vi "write-set.vi"(7 "dvr":refnum<data-value>, 8 "error in (no error)":errorcluster, 10 "y_axis":dbl[][](array[numeric]), 11 "x_axis":dbl[](array[numeric])) -> (0 "error out":errorcluster)   [LabVIEW 2015, in "lv-graph-global.lvlib"]
doc: "Preload can be used to store a data set in total. This can be used to \"load\" data from an alternate source rather than generating a set of points at a time."
uses:
  _controls/data.ctl
  _controls/configuration.ctl
  _controls/store_method.ctl
  lv-graph-global.lvlib
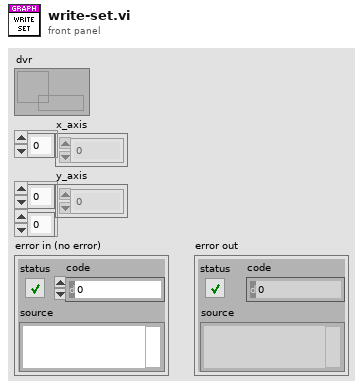
[diagram p1: front panel]
types:
  T1 = typedef "lv-graph-global.lvlib/data.ctl" = cluster{"configuration":T2, "index":i32, "x_axis":dbl[], "y_axis":dbl[][]}
  T2 = typedef "lv-graph-global.lvlib/configuration.ctl" = cluster{"store_method":T3, "rows":i32, "columns":i32}
  T3 = typedef "lv-graph-global.lvlib/store_method.ctl" = enum16{"<store_method>", "fixed", "grow"}
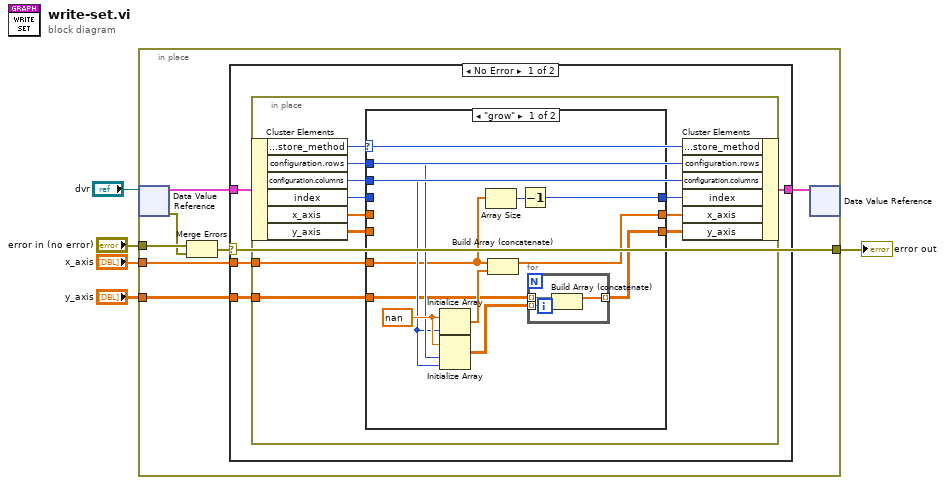
[diagram p0: block diagram]
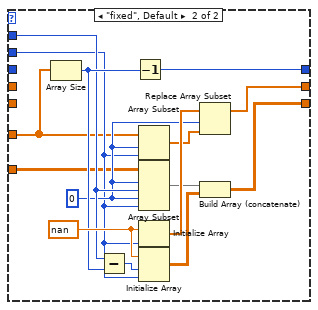
[diagram p2: hidden frame]
diagram:
  n1 = in-place {
    in-place-border: "error in (no error)" -> [w12]
    in-place-border: "x_axis" -> [w10]
    in-place-border: "y_axis" -> [w9]
    in-place-border: [w6] -> w1
    n2 = in-place-dvr #1("dvr") -> (w8:T1, w11:errorcluster)
    n3 = Merge Errors(w12, w11) -> (w6:errorcluster)
    n4 = case shown="No Error" w6 {
      tunnel: w10 -> [w16 _]
      tunnel: w9 -> [w15 _]
      tunnel: w8 -> [w14 w57]
      tunnel: [w13 w57] -> w7
      frame No Error {
        n5 = in-place {
          in-place-border: w16 -> [w27]
          in-place-border: w15 -> [w26]
          n6 = in-place-cluster #2(w14) -> ("configuration.store_method"=w25:T3, "configuration.rows"=w24:i32, "configuration.columns"=w23:i32, "index"=w22:i32, "x_axis"=w21:dbl[], "y_axis"=w20:dbl[][])
          n7 = case shown="\"grow\"" w25 {
            tunnel: w27 -> [w33 w46]
            tunnel: w26 -> [w31 w45]
            tunnel: w24 -> [w35 w49]
            tunnel: w23 -> [w34 w47]
            tunnel: w22 -> [_ _]
            tunnel: w21 -> [_ _]
            tunnel: w20 -> [_ _]
            tunnel: [w30 w44] -> w19
            tunnel: [w29 w43] -> w18
            tunnel: [w28 w42] -> w17
            frame "grow" {
              w37 = nan
              n8 = Initialize Array(w37, w34) -> (w36:dbl[])
              n9 = Initialize Array(w37, w35, w34) -> (w32:dbl[][])
              n10 = Array Size(array=w33) -> (size(s)=w38:i32)
              n11 = Build Array (concatenate)(w33, w36) -> (w29:dbl[])
              n12 = Decrement(x=w38) -> (x-1=w30:i32)
              n13 = for {
                tunnel: w31 -> [w41] mode=indexing
                tunnel: w32 -> [w40] mode=indexing
                tunnel: [w39] -> w28 mode=indexing
                n14 = Build Array (concatenate)(w41, w40) -> (w39:dbl[])
              }
            }
            frame "fixed", Default {
              w48 = 0 ("index")
              w56 = nan
              n15 = Array Size(array=w46) -> (size(s)=w53:i32)
              n16 = Subtract(x=w49, y=w53) -> (x-y=w52:i32)
              n17 = Decrement(x=w53) -> (x-1=w44:i32)
              n18 = Array Subset(array=w46, index=w48, length=w47) -> (w51:dbl[])
              n19 = Array Subset(array=w45, index (row)=w48, length (row)=w49, index (col)=w48, length (col)=w47) -> (w50:dbl[][])
              n20 = Initialize Array(w56, w47) -> (w55:dbl[])
              n21 = Initialize Array(w56, w52, w47) -> (w54:dbl[][])
              n22 = Replace Array Subset(array=w55, new element=w51, index=w48) -> (w43:dbl[])
              n23 = Build Array (concatenate)(w50, w54) -> (w42:dbl[][])
            }
          }
          n24 = in-place-cluster #2("configuration.store_method"=w25, "configuration.rows"=w24, "configuration.columns"=w23, "index"=w19, "x_axis"=w18, "y_axis"=w17) -> (w13:T1)
        }
      }
      frame Error {
      }
    }
    n25 = in-place-dvr #1(w7) -> ()  [unwired: 2 out]
  }
  "error out" <- w1
